vi "tls free.vi"(8 "error in":errorcluster, 11 "tls context":u64) -> (0 "error out":errorcluster)   [LabVIEW 2016, in "lv tls dll.lvlib"]
uses:
  lv tls dll.lvlib
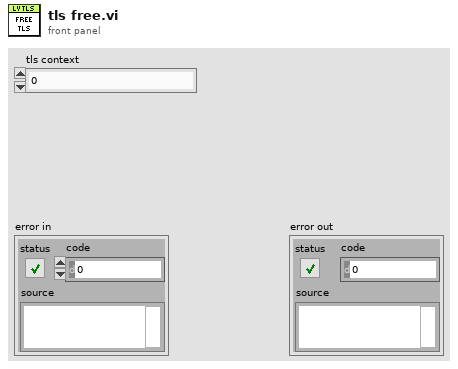
[diagram p1: front panel]
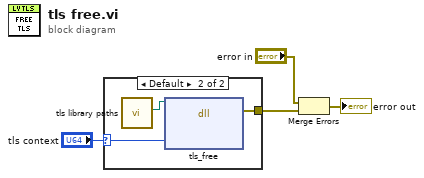
[diagram p0: block diagram]
diagram:
  n1 = case shown="Default" "tls context" {
    selector: "tls context" -> [_ w6]
    tunnel: [_ w5] -> w1
    frame 0 {
    }
    frame Default {
      n2 = call "tls library paths.vi"() -> ("libtls"=w7:path)  [unwired: 8 in, 3 out]
      n3 = dll-call lib="C:/Users/IEUser/Desktop/tlssimple/libtls-15.dll" fn="tls_free"(path in=w7, "context"=w6) -> (error out=w5:errorcluster)  [unwired: 4 in, 1 out]
    }
  }
  n4 = Merge Errors("error in", w1) -> (→"error out":errorcluster)
